vi "ticks_ms to mm_s.vi"(1 "ticks per ms":dbl) -> (0 "mm/s":dbl)   [LabVIEW 2017]
panel:
  in  "wheel dia (mm)":dbl=101.6
  in  "ticks per revolution":dbl=3200.0
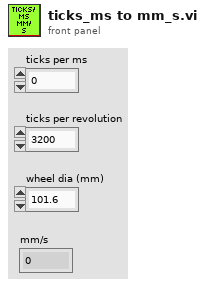
[diagram p1: front panel]
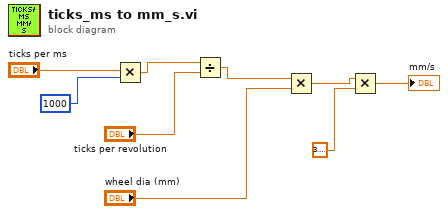
[diagram p0: block diagram]
diagram:
  n1 = Multiply(x="ticks per ms", y=1000) -> (x*y=w7:dbl)
  n2 = Divide(x=w7, y="ticks per revolution") -> (x/y=w5:dbl)
  n3 = Multiply(x=w5, y="wheel dia (mm)") -> (x*y=w2:dbl)
  n4 = Multiply(x=w2, y=3.141592653589793) -> (x*y=→"mm/s":dbl)
